vi "FestoCPX.DO.Data.States.Get.vi"(8 "error in (no error)":errorcluster, 10 "CPX.DO":T1[](array[typedef])) -> (0 "error out":errorcluster, 2 "State":bool[](array[boolean]))   [LabVIEW 2016]
uses:
  FestoCPX.DO.Signal.ctl
  FestoCPX.DO.Data.Fglb.Action.ctl
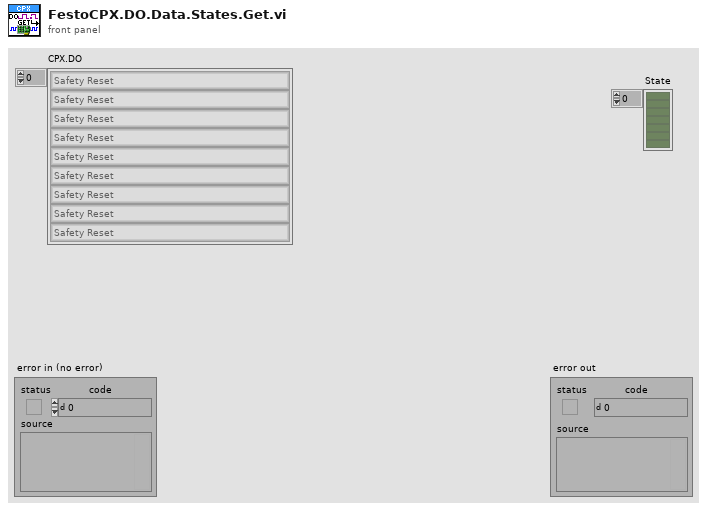
[diagram p1: front panel]
types:
  T1 = typedef "FestoCPX.DO.Signal.ctl" = enum16{"Safety Reset", "Air Main Valve", "Door Lock", "Button LED Start", "Button LED Stop", "Button LED Control", "Traffic LED Red", "Traffic LED Orange", "Traffic LED Green", "Horn", "Laser Interlock", "Laser Trigger", "Laser Fume Extractor", "Product Suction Gripper Slot 1 A", "Product Suction Gripper Slot 1 B", "Product Suction Gripper Slot 2 A", "Product Suction Gripper Slot 2 B", "Product Suction Gripper Slot 3 A", "Product Suction Gripper Slot 3 B", "Product Suction Gripper Slot 4 A", "Product Suction Gripper Slot 4 B", "Product Suction Gripper Final A", "Product Suction Gripper Final B", "Lamp", "Q1 Product Move Work", "Q1 Product Move Home", "Q2 Table Turn Work", "Q2 Table Turn Home", "Q3 Product Lift A", "Q3 Product Lift B", "Q4 Product Arm OK", "Q4 Product Arm NOK", "Q5 Product Arm Work", "Q6 Product BlowOut A", "Q6 Product BlowOut B"}
  T2 = typedef "FestoCPX.DO.Data.Fglb.Action.ctl" = enum16{"init", "set", "get", "check", "select", "reset"}
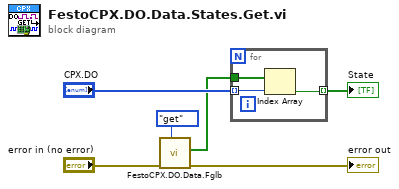
[diagram p0: block diagram]
diagram:
  n1 = call "FestoCPX.DO.Data.Fglb.vi"("state (get all)"=FestoCPX.DO.Data.Fglb.Action."get", "error in (no error)"="error in (no error)") -> ("error out"=→"error out":errorcluster, "State out"=w1:bool[])  [unwired: 7 in, 1 out]
  n2 = for {
    tunnel: w1 -> [w9]
    tunnel: "CPX.DO" -> [w8] mode=indexing
    tunnel: [w7] -> w5 mode=indexing
    n3 = Index Array(array=w9, index=w8) -> (element=w7:bool)
  }
  "State" <- w5
